vi "调用子VI并弹出界面.vi"() -> ()   [LabVIEW 2017]
panel:
  in  "停止":bool
  in  "?":bool
  out "Result":dbl
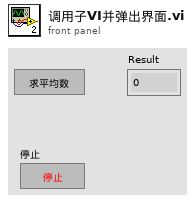
[diagram p1: front panel]
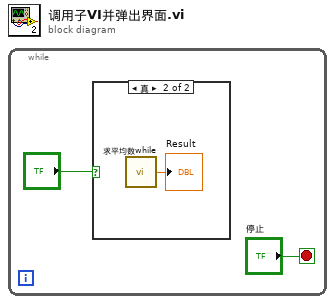
[diagram p0: block diagram]
diagram:
  n1 = while {
    stop <- "停止" stop-if-true
    n2 = case shown="真" "?" {
      frame False {
      }
      frame True {
        n3 = call "求平均数while.vi"() -> ("Result"=→"Result":dbl)  [unwired: 2 in]
      }
    }
  }
